vi "Write_Line_To_Command_List.vi"(0 "Byte Stream File in":refnum<file>, 1 "P6":dbl, 2 "Step":i32, 3 "P5":dbl, 4 "P1":dbl, 6 "Include Step":bool, 7 "CmdNumb":i32, 8 "P7":dbl, 9 "P2":dbl, 10 "Comment":string, 11 "P3":dbl, 13 "P4":dbl) -> (14 "Byte Stream File out":refnum<file>)   [LabVIEW 2018]
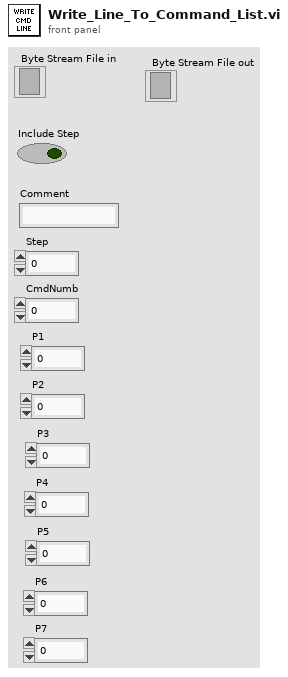
[diagram p1: front panel]
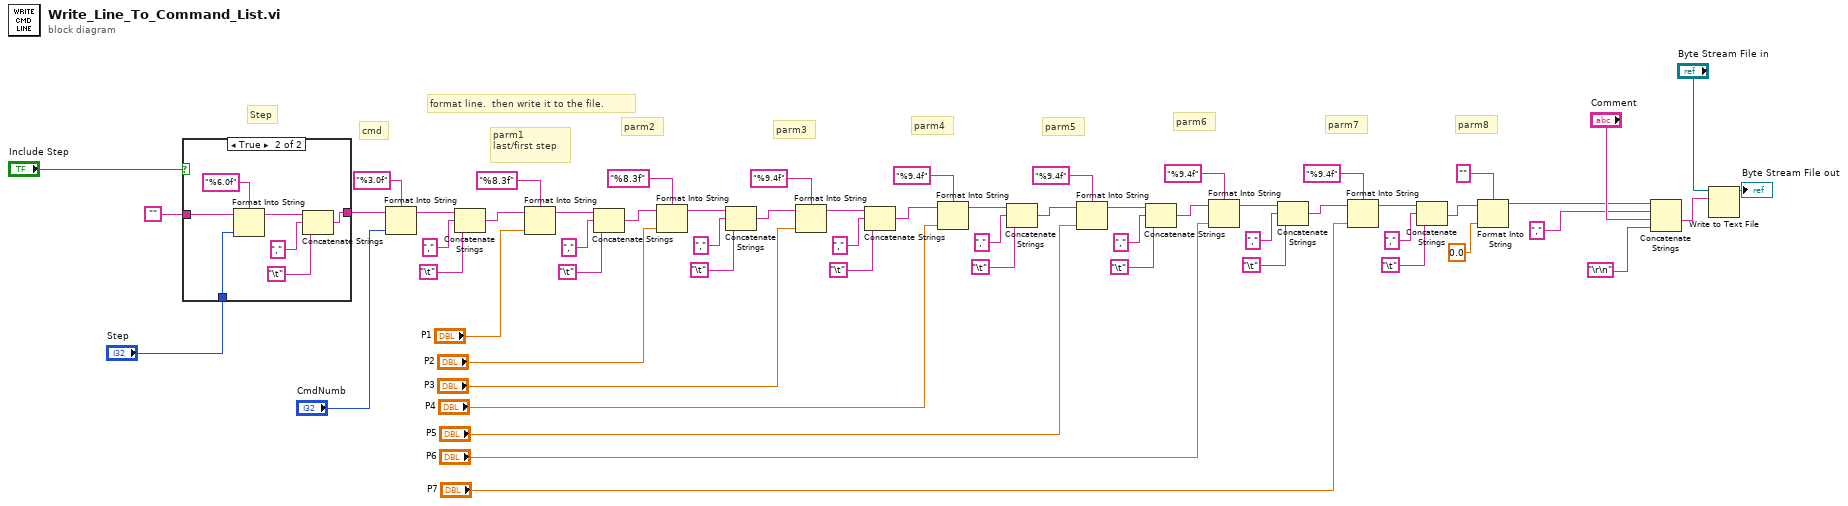
[diagram p0: block diagram]
diagram:
  # "format line.  then write it to the file."
  # "parm8"
  # "parm7"
  # "parm6"
  # "parm5"
  # "parm4"
  # "parm3"
  # "parm2"
  # "parm1\nlast/first step"
  # "cmd"
  # "Step"
  n1 = case shown="True" "Include Step" {
    tunnel: "" -> [w62 w66]
    tunnel: "Step" -> [_ w65]
    tunnel: [w62 w63] -> w9
    frame False {
    }
    frame True {
      n2 = Format Into String(format string="%6.0f", initial string=w66, w65) -> (resulting string=w69:string)  [unwired: 1 in, 1 out]
      n3 = Concatenate Strings(w69, "," ("string"), "\t") -> (w63:string)
    }
  }
  n4 = Format Into String(format string="%3.0f", initial string=w9, "CmdNumb") -> (resulting string=w5:string)  [unwired: 1 in, 1 out]
  n5 = Concatenate Strings(w5, "," ("string"), "\t") -> (w14:string)
  n6 = Format Into String(format string="%8.3f", initial string=w14, "P1") -> (resulting string=w10:string)  [unwired: 1 in, 1 out]
  n7 = Concatenate Strings(w10, "," ("string"), "\t") -> (w24:string)
  n8 = Format Into String(format string="%8.3f", initial string=w24, "P2") -> (resulting string=w15:string)  [unwired: 1 in, 1 out]
  n9 = Concatenate Strings(w15, "," ("string"), "\t") -> (w23:string)
  n10 = Format Into String(format string="%9.4f", initial string=w23, "P3") -> (resulting string=w19:string)  [unwired: 1 in, 1 out]
  n11 = Concatenate Strings(w19, "," ("string"), "\t") -> (w44:string)
  n12 = Format Into String(format string="%9.4f", initial string=w44, "P4") -> (resulting string=w25:string)  [unwired: 1 in, 1 out]
  n13 = Concatenate Strings(w25, "," ("string"), "\t") -> (w33:string)
  n14 = Format Into String(format string="%9.4f", initial string=w33, "P5") -> (resulting string=w29:string)  [unwired: 1 in, 1 out]
  n15 = Concatenate Strings(w29, "," ("string"), "\t") -> (w43:string)
  n16 = Format Into String(format string="%9.4f", initial string=w43, "P6") -> (resulting string=w34:string)  [unwired: 1 in, 1 out]
  n17 = Concatenate Strings(w34, "," ("string"), "\t") -> (w42:string)
  n18 = Format Into String(format string="%9.4f", initial string=w42, "P7") -> (resulting string=w38:string)  [unwired: 1 in, 1 out]
  n19 = Concatenate Strings(w38, "," ("string"), "\t") -> (w46:string)
  n20 = Format Into String(format string="", initial string=w46, 0.0 ("input 1")) -> (resulting string=w47:string)  [unwired: 1 in, 1 out]
  n21 = Concatenate Strings(w47, "," ("string"), "Comment", "\r\n") -> (w57:string)
  n22 = Write to Text File(file (use dialog)="Byte Stream File in", text=w57) -> (refnum out=→"Byte Stream File out":refnum<file>)  [unwired: 2 in, 2 out]
